vi "Write SubPanel Ref.vi"(8 "error in (no error)":errorcluster, 10 "SubPanel Ref":refnum<vi>, 11 "Instrument Finder in":refnum<class "Instrument Finder.lvclass">) -> (0 "error out":errorcluster, 3 "Instrument Finder out":refnum<class "Instrument Finder.lvclass">)   [LabVIEW 2014]
uses:
  Instrument Finder.lvclass
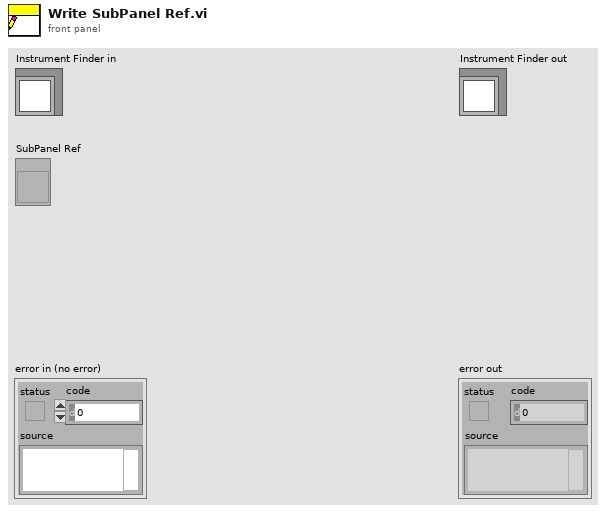
[diagram p1: front panel]
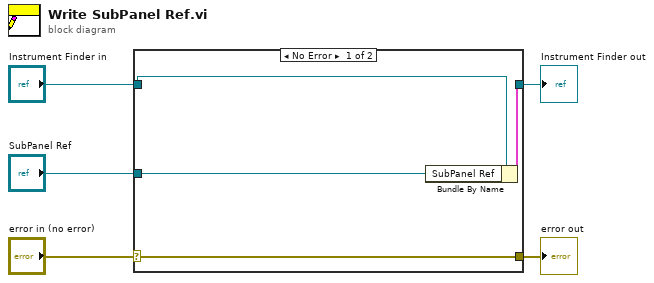
[diagram p0: block diagram]
diagram:
  n1 = case shown="No Error" "error in (no error)" {
    selector: "error in (no error)" -> [w9 w10]
    tunnel: [w9 w10] -> w4
    tunnel: [w7 w11] -> w2
    tunnel: "Instrument Finder in" -> [w8 w11]
    tunnel: "SubPanel Ref" -> [w6 _]
    frame No Error {
      n2 = Bundle By Name(cluster=w8, "SubPanel Ref"=w6) -> (w7:cluster{})
    }
    frame Error {
    }
  }
  "error out" <- w4
  "Instrument Finder out" <- w2
